vi "while loop with random number.vi"() -> ()   [LabVIEW 2018]
panel:
  out "number (0 to 1)":dbl
  out "Numeric":i32
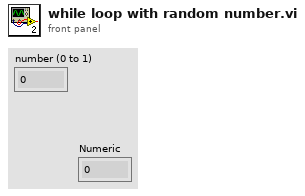
[diagram p1: front panel]
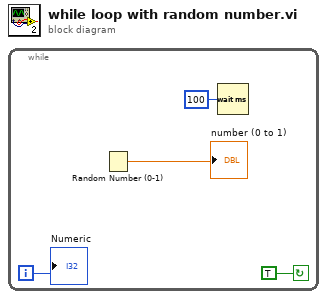
[diagram p0: block diagram]
diagram:
  n1 = while {
    i -> [w3]
    stop <- TRUE continue-if-true
    n2 = Random Number (0-1)() -> (number: 0 to 1=→"number (0 to 1)":dbl)
    n3 = Wait (ms)(milliseconds to wait=u32 100) -> ()  [unwired: 1 out]
    "Numeric" <- w3
  }
